vi "Get Channels from Section.vi"(7 "channel by GUID":bool, 8 "error in":errorcluster, 9 "channel array names":string[](array[string]), 10 "GUID section":string, 11 "custom device ref in":T1 format="%.0x") -> (0 "error out":errorcluster, 1 "channel array refs out":T1[](array[typedef]) format="%.0x", 2 "section ref out":T1 format="%.0x", 3 "custom device ref out":T1 format="%.0x", 4 "all channels found?":bool, 6 "session found?":bool)   [LabVIEW 2020, in "AIM ARINC 664 Scripting.lvlib"]
uses:
  AIM ARINC 664 Scripting.lvlib
  <vilib>/NI VeriStand/Custom Device API/Custom Device Item Ref.ctl
  <vilib>/NI VeriStand/Custom Device Tools/Custom Device Utility Library/NI VeriStand - Search for Item by GUID.vi
  <vilib>/NI VeriStand/Custom Device Tools/Custom Device Utility Library/NI VeriStand - Search for All Items by GUID.vi
  <vilib>/NI VeriStand/Custom Device Tools/Custom Device Utility Library/NI VeriStand - Search for Item by Name.vi
  <vilib>/NI VeriStand/Custom Device Tools/Custom Device Utility Library/Custom Device Utility Library.lvlib
  <vilib>/NI VeriStand/Custom Device API/Custom Device API.lvlib
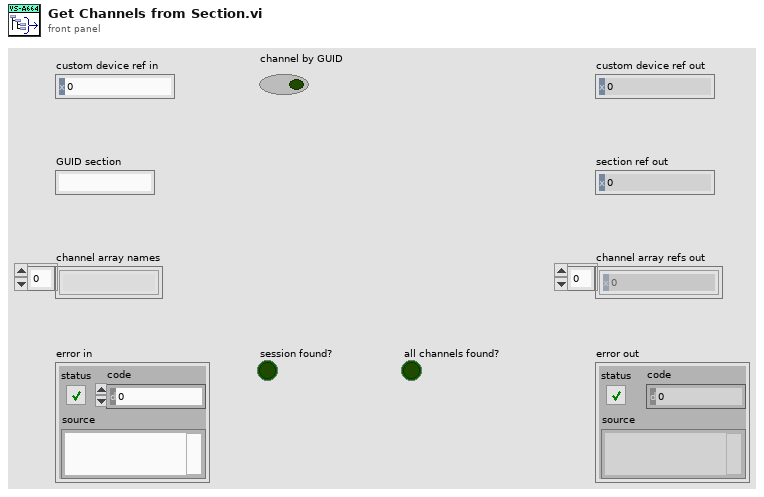
[diagram p1: front panel]
types:
  T1 = typedef "Custom Device API.lvlib/Custom Device Item Ref.ctl" = u64
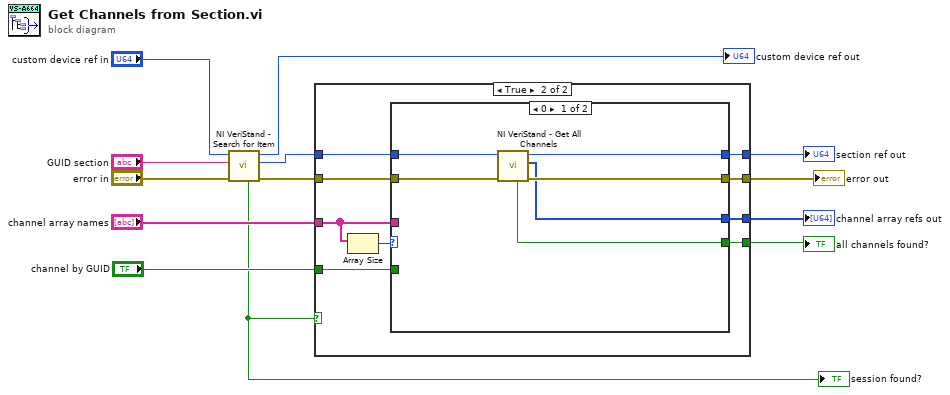
[diagram p0: block diagram]
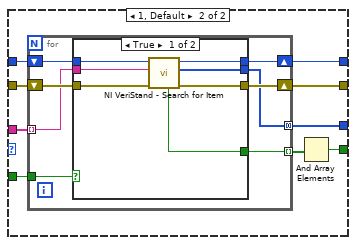
[diagram p3: hidden frame]
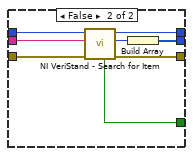
[diagram p4: hidden frame]
diagram:
  n1 = call-poly <vilib>:"NI VeriStand - Search for Item.vi"("error in"="error in", "Item GUID"="GUID section", "Section Ref in"="custom device ref in") -> ("error out"=w11:errorcluster, "Item Ref"=w12:T1, "Section Ref out"=→"custom device ref out":T1, "Found"=w1:bool)  [unwired: 5 in]
  "session found?" <- w1
  n2 = case shown="True" w1 {
    selector: w1 -> [w14 _]
    tunnel: w12 -> [w16 w25]
    tunnel: w11 -> [w15 w24]
    tunnel: "channel array names" -> [_ w23]
    tunnel: [w14 w21] -> w7
    tunnel: [w15 w20] -> w6
    tunnel: [_ w19] -> w5
    tunnel: [w16 w18] -> w4
    tunnel: "channel by GUID" -> [_ w17]
    frame False {
    }
    frame True {
      n3 = Array Size(array=w23) -> (size(s)=w22:i32)
      n4 = case shown="0" w22 {
        tunnel: [w26 w40] -> w19
        tunnel: [w28 w39] -> w20
        tunnel: w25 -> [w31 w38]
        tunnel: [w30 w37] -> w18
        tunnel: w24 -> [w29 w36]
        tunnel: w23 -> [_ w35]
        tunnel: [w27 w33] -> w21
        tunnel: w17 -> [_ w32]
        frame 0 {
          n5 = call <vilib>:"NI VeriStand - Get All Channels.vi"("error in"=w29, "Section Ref in"=w31) -> ("error out"=w28:errorcluster, "Channel Refs"=w26:T1[], "Section Ref out"=w30:T1, "Found"=w27:bool)  [unwired: 6 in]
        }
        frame 1, Default {
          n6 = for {
            tunnel: [w44] -> w40 mode=concatenating
            shift-right: [w45] -> w39
            shift-left: w36 -> [w48]
            tunnel: w35 -> [w43] mode=indexing
            shift-right: [w47] -> w37
            shift-left: w38 -> [w46]
            tunnel: [w42] -> w34 mode=indexing
            tunnel: w32 -> [w41]
            n7 = case shown="True" w41 {
              tunnel: w48 -> [w55 w63]
              tunnel: [w54 w62] -> w47
              tunnel: w46 -> [w53 w61]
              tunnel: [w52 w60] -> w45
              tunnel: [w51 w56] -> w44
              tunnel: w43 -> [w50 w58]
              tunnel: [w49 w57] -> w42
              frame True {
                n8 = call-poly <vilib>:"NI VeriStand - Search for Item.vi"("error in"=w55, "Item GUID"=w50, "Section Ref in"=w53) -> ("error out"=w52:errorcluster, "Item Refs"=w51:T1[], "Section Ref out"=w54:T1, "Found"=w49:bool)  [unwired: 5 in]
              }
              frame False {
                n9 = call-poly <vilib>:"NI VeriStand - Search for Item.vi"("error in"=w63, "Item Name"=w58, "Section Ref in"=w61) -> ("error out"=w60:errorcluster, "Item Ref"=w59:T1, "Section Ref out"=w62:T1, "Found"=w57:bool)  [unwired: 5 in]
                n10 = Build Array(w59) -> (w56:T1[])
              }
            }
          }
          n11 = And Array Elements(Boolean array=w34) -> (logical AND=w33:bool)
        }
      }
    }
  }
  "all channels found?" <- w7
  "channel array refs out" <- w5
  "error out" <- w6
  "section ref out" <- w4
